vi "Process.vi"(8 "error in":errorcluster, 11 "Inst.TC":refnum<class "Inst.TC.lvclass">) -> (0 "error out":errorcluster, 3 "Inst.TC out":refnum<class "Inst.TC.lvclass">)   [LabVIEW 2019, in "Inst.TC.lvclass"]
doc: "---------------------------------------------------------------\nJKI State Machine Objects™\nhttp://jki.net/state-machine-objects/\nCopyright (C) 2005-2015, JKI <info@jki.net>\nALL RIGHTS RESERVED"
uses:
  Inst.TC.lvclass
  <vilib>/JKI/JKI SMO/SMO/SMO.lvclass
  <userlib>/LevyLab/RemoteControl/RemoteControl/Typedefs/Message--Cluster.ctl
  <userlib>/LevyLab/RemoteControl/RemoteControl/RemoteControl.lvclass
  Typedefs/PrivateEvents--Inst.TC.MessageToProcess.ctl
  C:/Program Files/National Instruments/LabVIEW 2019/user.lib/LevyLab/Instrument Framework/Instrument Types/Cryostat/Instrument.Cryostat.lvclass
  C:/Program Files/National Instruments/LabVIEW 2019/user.lib/LevyLab/Instrument Framework/Instrument/Instrument.lvclass
  C:/Program Files/National Instruments/LabVIEW 2019/vi.lib/JKI/JKI SMO/SMO/SMO.lvclass
  <userlib>/LevyLab/Instrument Framework/Instrument/Instrument.lvclass
  <userlib>/LevyLab/Instrument Framework/Instrument Types/Cryostat/Instrument.Cryostat.lvclass
  <userlib>/LevyLab/Instrument Framework/Instrument/API/Instrument.sendMessageToProcess (variant).vi
  <userlib>/LevyLab/Debug/Debug.lvlib
panel:
  out "Status":string
  out "State History":string
  # "Inst.TC"
  # "Inst.TC"
  # "For instructions on how to use the JKI State Machine Objects, examples and video tutorials, visit:\nhttp://jki.net/state-machine-objects/\n\nJKI State Machine Objects™\nhttp://jki.net/state-machine-objects/\nCopyright (C) 2005-2015, JKI <info@jki.net>\nALL RIGHTS RESERVED"
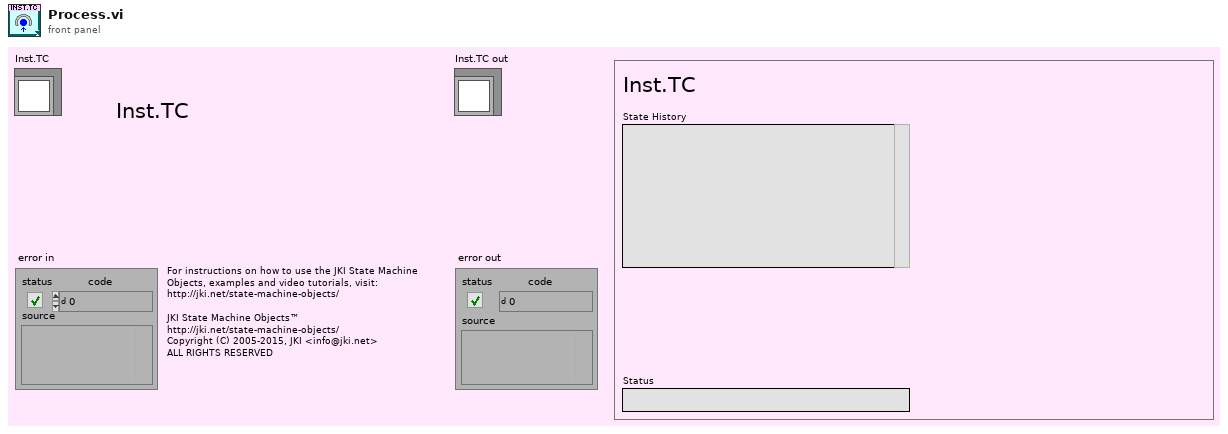
[diagram p1: front panel]
types:
  T1 = enum32{"invalid app kind", "Development System", "Run Time System", "Student Edition", "Embedded LabVIEW", "Evaluation", "Custom"}
  T2 = enum32{"Invalid", "Standard", "Closed", "Hidden", "Minimized", "Maximized"}
  T3 = typedef "RemoteControl.lvlib/RemoteControl.lvclass/Message--Cluster.ctl" = cluster{"Command":string, "Data":variant, "ID":string, "error":errorcluster}
  T4 = typedef "Inst.TC.lvclass/PrivateEvents--Inst.TC.MessageToProcess.ctl" = cluster{"Message":T3}
  T5 = cluster{"Core":cluster{"Current VI Reference":refnum<vi>, "Close Panel on Exit?":bool, "Last Error":cluster{"error":errorcluster, "previous state":string, "remaining states":string}, "Shutdown?":bool}, "SMO":refnum<class "Inst.TC.lvclass">, "Running Step":i32, "sequence":string[], "MessageToProcess":T4}
  T6 = cluster{"Current VI Reference":refnum<vi>, "Close Panel on Exit?":bool, "Last Error":cluster{"error":errorcluster, "previous state":string, "remaining states":string}, "Shutdown?":bool}
  T7 = typedef "SMO.lvclass/Protected Events.ctl" = cluster{"StopProcesses":refnum<user-event>, "AbortProcesses":refnum<user-event>, "Config Changed":refnum<user-event>, "Dependency":refnum<user-event>}
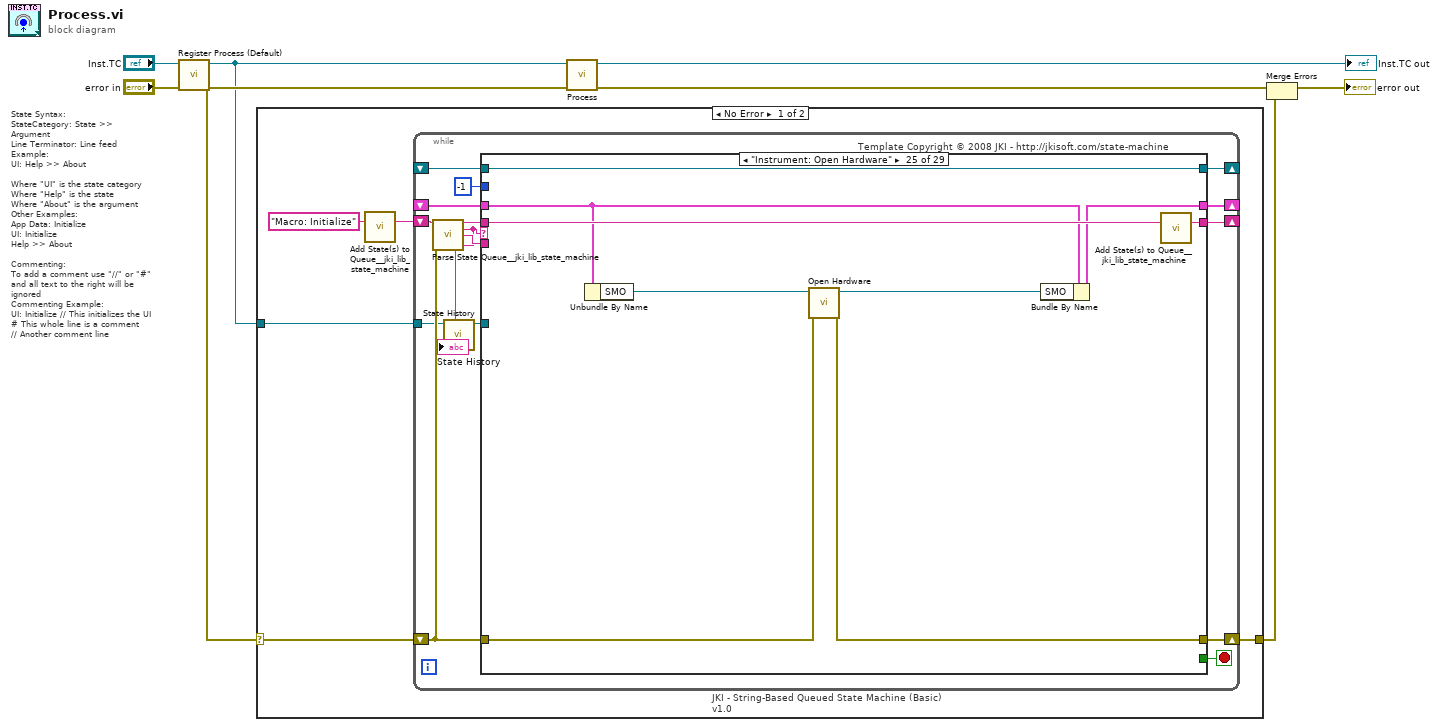
[diagram p0: block diagram]
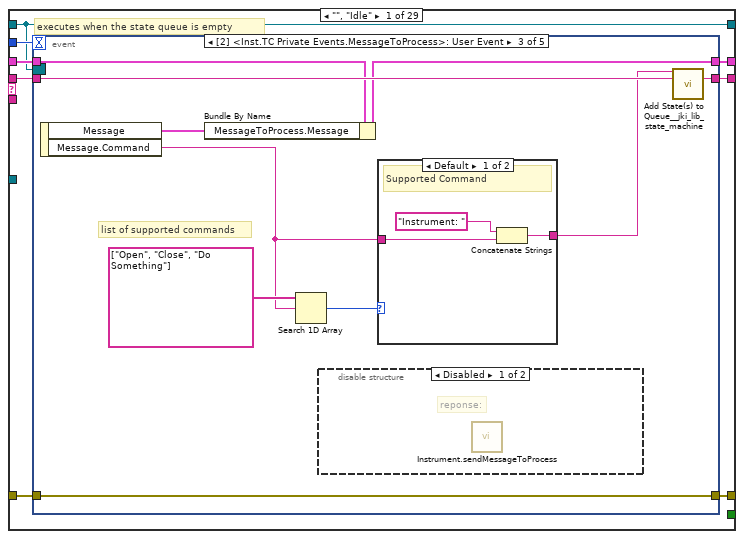
[diagram p2: hidden frame]
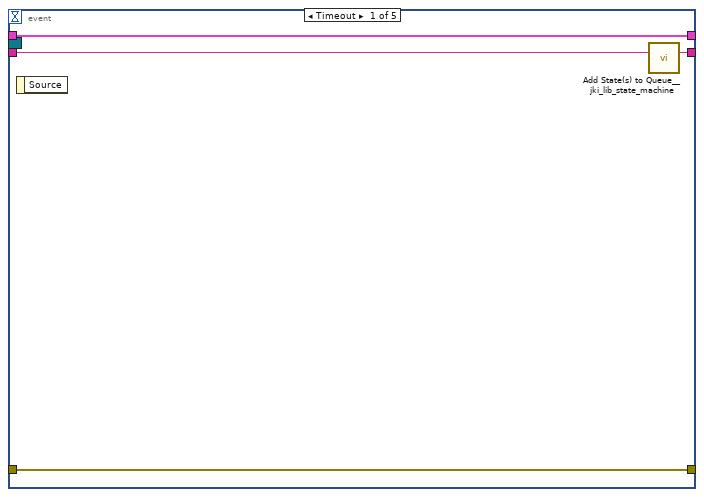
[diagram p3: hidden frame]
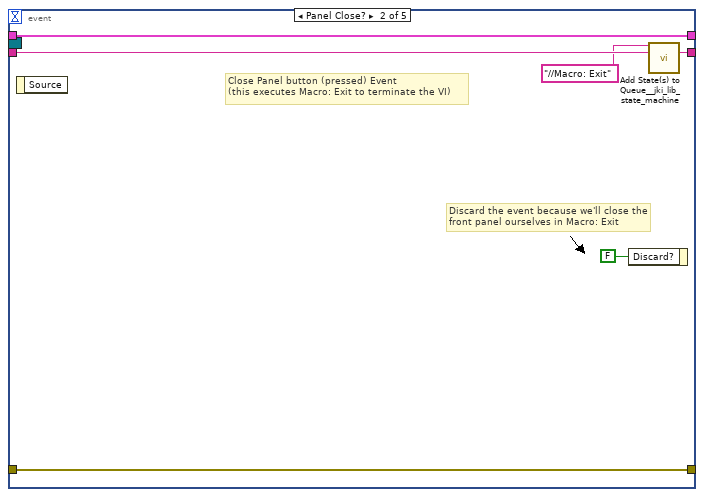
[diagram p4: hidden frame]
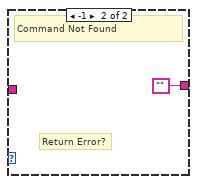
[diagram p6: hidden frame]
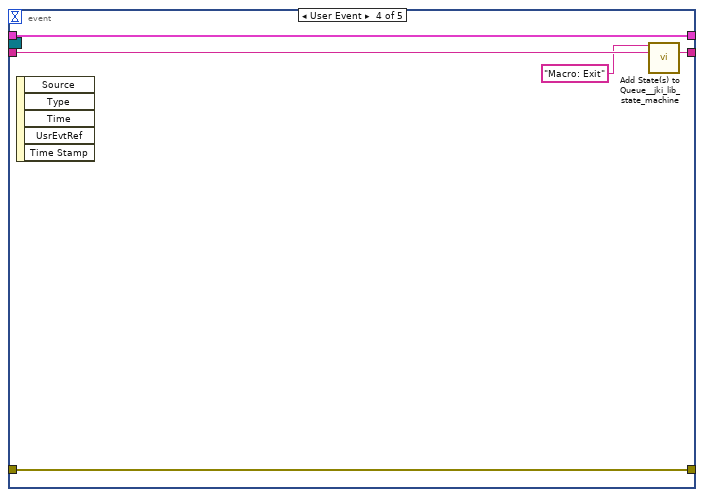
[diagram p7: hidden frame]
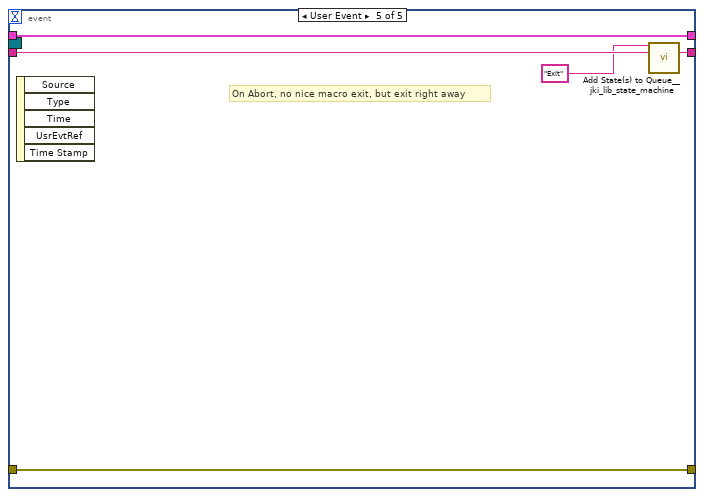
[diagram p8: hidden frame]
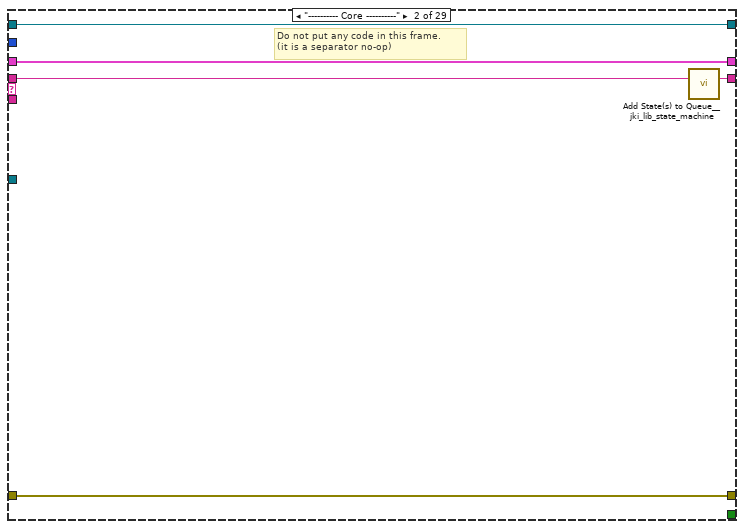
[diagram p9: hidden frame]
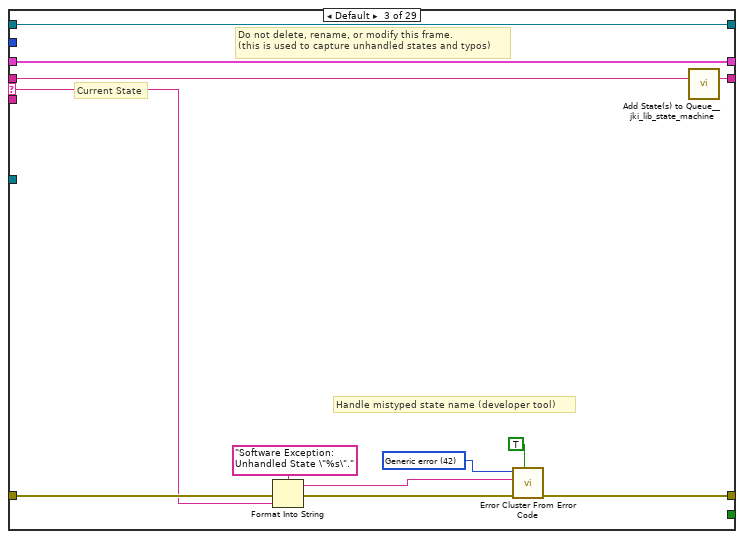
[diagram p10: hidden frame]
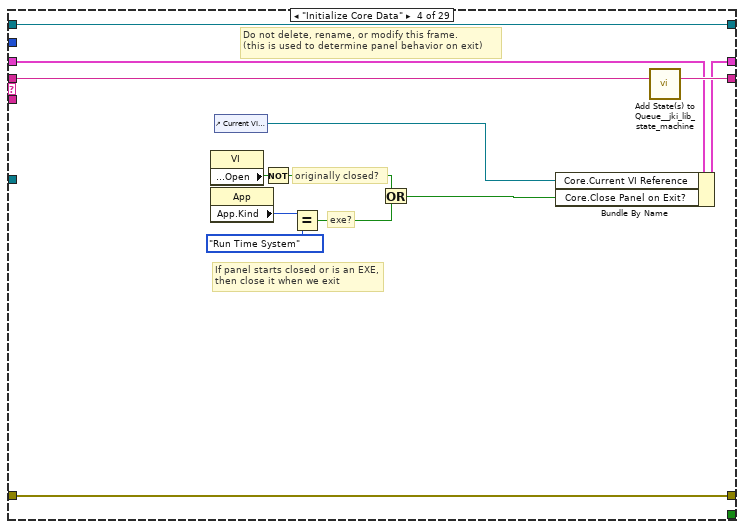
[diagram p11: hidden frame]
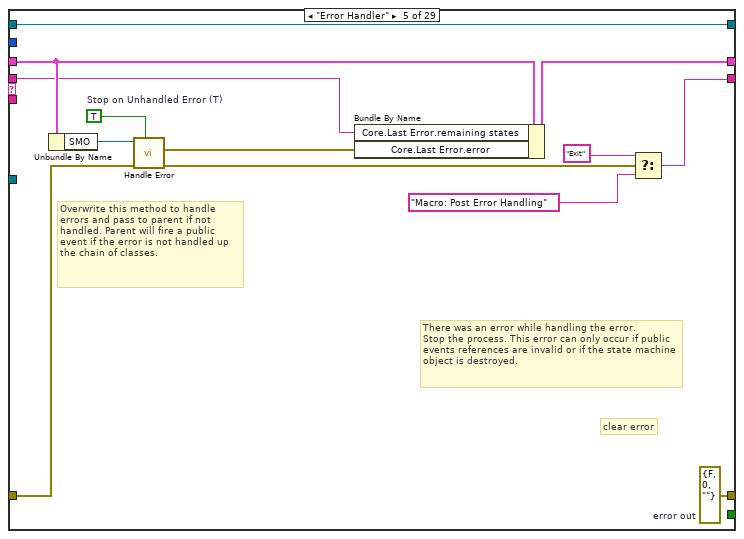
[diagram p12: hidden frame]
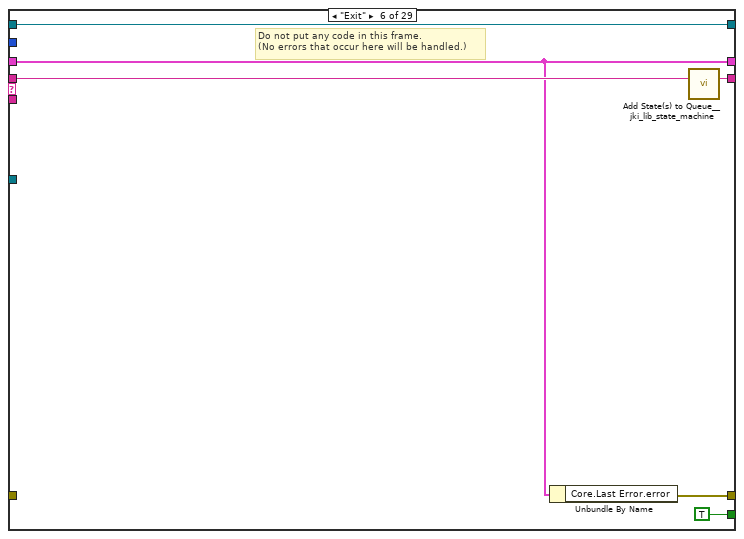
[diagram p13: hidden frame]
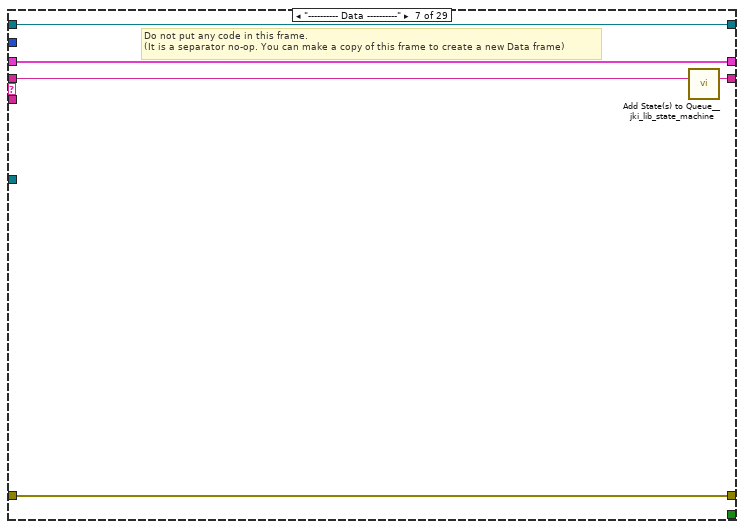
[diagram p14: hidden frame]
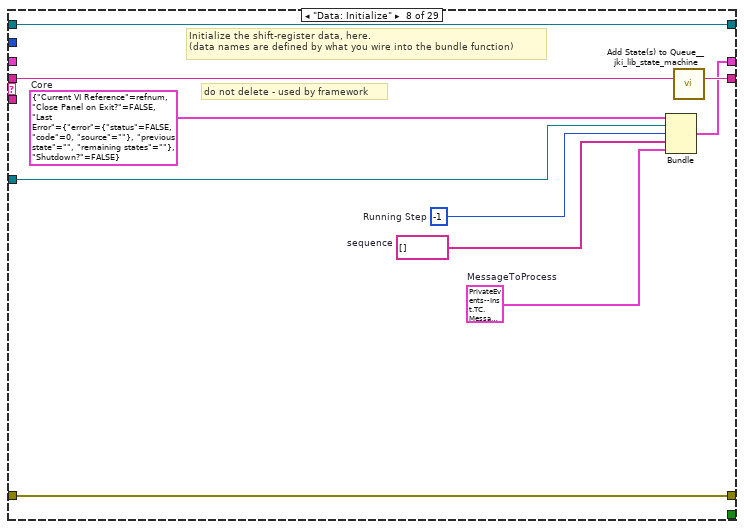
[diagram p15: hidden frame]
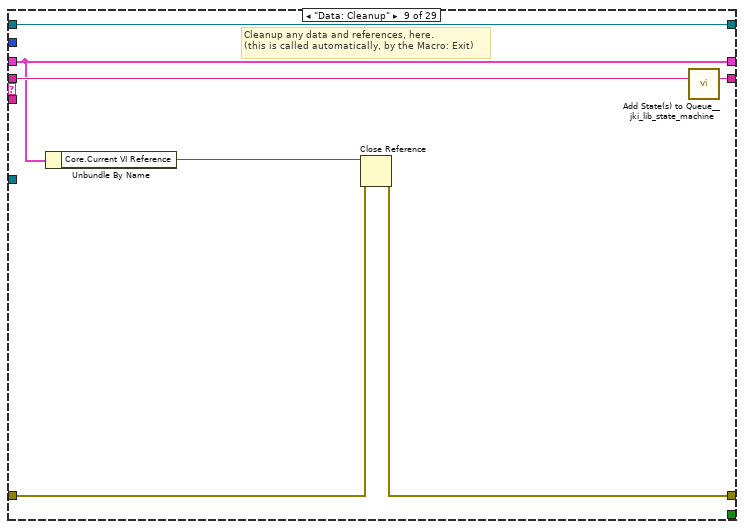
[diagram p16: hidden frame]
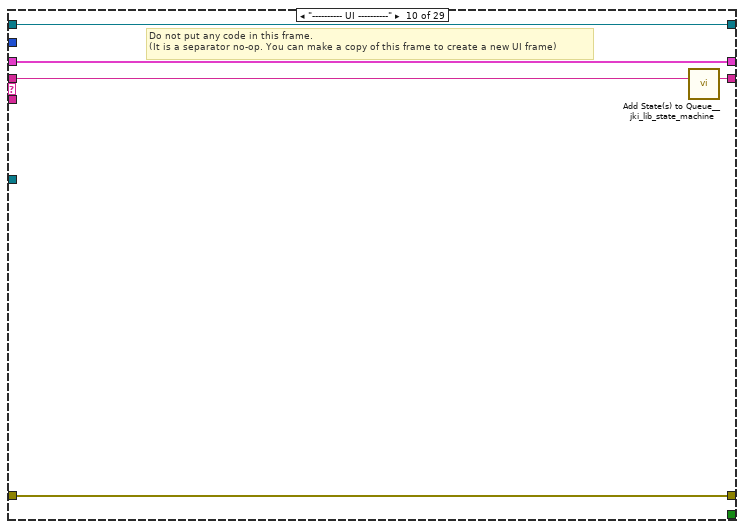
[diagram p17: hidden frame]
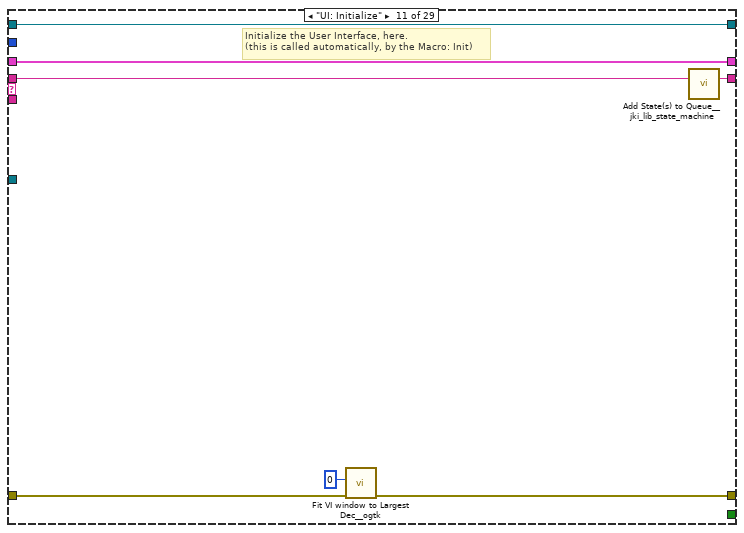
[diagram p18: hidden frame]
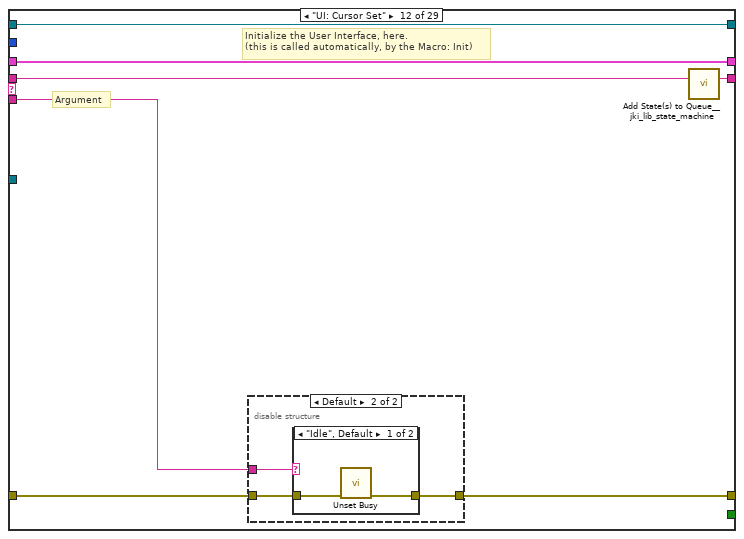
[diagram p19: hidden frame]
diagram:
  # "State Syntax:\nStateCategory: State >> Argument\nLine Terminator: Line feed\nExample:\nUI: Help >> About\n\nWhere \"UI\" is the state category\nWhere \"Help\" is the state\nWhere \"About\" is the argument\nOther Examples:\nApp Data: Initialize\nUI: Initialize\nHelp >> About\n\nCommenting:\nTo add a comment use \"//\" or \"#\" and all text to the right will be ignored\nCommenting Example:\nUI: Initialize // This initializes the UI\n# This whole line is a comment\n// Another comment line"
  n1 = call <vilib>:"Register Process (Default).vi"("error in (no error)"="error in", "SMO"="Inst.TC") -> ("error out"=w5:errorcluster, "SelfRef"=w4:refnum<class "Inst.TC.lvclass">)  [unwired: 8 in]
  n2 = case shown="No Error" w5 {
    selector: w5 -> [w10 w379]
    tunnel: w4 -> [w11 _]
    tunnel: [w9 w379] -> w1
    frame No Error {
      n3 = call <vilib>:"Add State(s) to Queue__jki_lib_state_machine.vi"("State(s) in (\"\")"="Macro: Initialize") -> ("States Out"=w13:string)  [unwired: 14 in]
      n4 = while "JKI - String-Based Queued State Machine (Basic) v1.0" {
        shift-right: [w23] -> _
        shift-left: _ -> [w22]
        shift-right: [w26] -> w9
        shift-left: w10 -> [w20]
        shift-right: [w25] -> _
        shift-left: w13 -> [w27]
        tunnel: w11 -> [w14]
        shift-right: [w19] -> _
        shift-left: _ -> [w18]
        stop <- w24 stop-if-true
        # "Template Copyright © 2008 JKI - http://jkisoft.com/state-machine"
        n5 = call <vilib>:"Parse State Queue__jki_lib_state_machine.vi"("State Queue"=w27, "Error In (no error)"=w20) -> ("Remaining States"=w29:string, "Current State"=w17:string, "Arguments"=w28:string)  [unwired: 11 in]
        n6 = call <userlib>:"State History.vi"("Current State"=w17, "SMO"=w14) -> ("SMO"=w15:refnum<class "Inst.TC.lvclass">, "History"=→"State History":string)  [unwired: 8 in]
        n7 = case shown="\"Instrument: Open Hardware\"" w17 {
          selector: w17 -> [_ _ w78 _ _ _ _ _ _ _ _ _ _ _ _ _ _ _ _ _ _ _ _ _ _ _ _ _ _]
          tunnel: w29 -> [w37 w76 w82 w101 w106 w120 w125 w135 w142 w147 w154 w161 w177 w209 w228 w240 w261 w283 w288 w299 w304 w317 w323 w330 w339 w348 w353 w359 w378]
          tunnel: w28 -> [_ _ _ _ _ _ _ _ _ _ _ w155 w171 _ _ _ _ _ _ _ _ _ _ _ _ _ _ w354 w362]
          tunnel: w22 -> [w35 w73 w80 w92 w110 w116 w122 _ w137 w144 w152 w159 w173 w206 w225 w230 w251 w264 w285 w296 w301 w310 w321 w325 w335 w344 w349 w355 w368]
          tunnel: [w34 w74 w84 w98 w111 w115 w123 w127 w138 w145 w149 w156 w174 w207 w213 w238 w259 w266 w286 w290 w302 w313 w319 w327 w332 w341 w350 w356 w370] -> w26
          tunnel: w20 -> [w33 w74 w83 w98 w112 _ w123 w127 w139 w145 w148 w157 w175 w207 w217 w238 w259 w267 w286 w291 w302 w307 w319 w327 w331 w340 w350 w356 w364]
          tunnel: [w36 w75 w81 w100 w102 w119 w124 w134 w141 w146 w153 w160 w176 w208 w227 w239 w260 w282 w287 w298 w303 w316 w322 w329 w338 w347 w352 w358 w377] -> w25
          tunnel: [_ _ _ _ _ TRUE _ _ _ _ _ _ _ _ _ _ _ _ _ _ _ _ _ _ _ _ _ _ _] -> w24
          tunnel: [w32 w73 w80 w99 w109 w116 w122 w133 w137 w144 w152 w159 w173 w206 w225 w231 w252 w264 w285 w296 w301 w310 w321 w326 w336 w345 w349 w355 w367] -> w23
          tunnel: -1 ("Timeout") -> [w31 _ _ _ _ _ _ _ _ _ _ _ _ _ _ _ _ _ _ _ _ _ _ _ _ _ _ _ _]
          tunnel: w15 -> [_ _ _ _ _ _ _ w128 _ _ _ _ _ _ w221 _ _ w263 _ _ _ _ _ _ _ _ _ _ _]
          tunnel: [w30 w72 w77 w89 w114 w117 w121 w132 w136 w143 w151 w158 w170 w205 w226 w237 w258 w277 w284 w297 w300 w315 w320 w328 w337 w346 w351 w357 w376] -> w19
          tunnel: w18 -> [w30 w72 w77 w89 w114 w117 w121 w132 w136 w143 w151 w158 w170 w205 w226 w237 w258 w277 w284 w297 w300 _ w320 w328 w337 w346 w351 w357 w376]
          frame "", "Idle" {
            # "executes when the state queue is empty"
            n8 = event shown="[2] <Inst.TC Private Events.MessageToProcess>: User Event" {
              selector: w30 -> [_ _ _ _ _]
              dyn-events: _ -> [_ _ _ _ _]
              timeout: w31 -> [_ _ _ _ _]
              tunnel: w37 -> [w41 w47 w57 w66 w71]
              tunnel: [w40 w46 w56 w65 w70] -> w36
              tunnel: w35 -> [w38 w44 w49 w63 w68]
              tunnel: [w39 w45 w55 w64 w69] -> w34
              tunnel: w33 -> [w39 w45 w55 w64 w69]
              tunnel: [w38 w44 w50 w63 w68] -> w32
              event Timeout {
                n9 = event-data() -> ()  [unwired: 1 in, 1 out]
                n10 = call <vilib>:"Add State(s) to Queue__jki_lib_state_machine.vi"("State(s) in (\"\")"=w41) -> ("States Out"=w40:string)  [unwired: 14 in]
              }
              event Panel Close? {
                # "Discard the event because we'll close the front panel ourselves in Macro: Exit"
                # "Close Panel button (pressed) Event\n(this executes Macro: Exit to terminate the VI)"
                n11 = event-data() -> ()  [unwired: 1 in, 1 out]
                n12 = event-data("Discard?"=FALSE) -> ()  [unwired: 1 in, 1 out]
                n13 = call <vilib>:"Add State(s) to Queue__jki_lib_state_machine.vi"("State(s) in Front (\"\")"="//Macro: Exit", "State(s) in (\"\")"=w47) -> ("States Out"=w46:string)  [unwired: 13 in]
              }
              event User Event {
                # "list of supported commands"
                n14 = event-data() -> ("Message"=w48:T3, "Message.Command"=w51:string)  [unwired: 1 in]
                n15 = Bundle By Name(cluster=w49, "MessageToProcess.Message"=w48) -> (w50:T5)
                n16 = Search 1D Array(1D array=string[] ["Open", "Close", "Do Something"], element=w51) -> (index of element=w54:i32)  [unwired: 1 in]
                n17 = disable-structure shown="Disabled" {
                  frame Disabled {
                    # "reponse:"
                    n18 = call-poly <userlib>:"Instrument.sendMessageToProcess.vi"() -> ()  [unwired: 10 in, 2 out]
                  }
                  frame Enabled {
                  }
                }
                n19 = case shown="Default" w54 {
                  tunnel: [w60 "" ("Empty String Constant")] -> w52
                  tunnel: w51 -> [w59 _]
                  frame Default {
                    # "Supported Command"
                    n20 = Concatenate Strings("Instrument: ", w59) -> (w60:string)
                  }
                  frame -1 {
                    # "Return Error?"
                    # "Command Not Found"
                  }
                }
                n21 = call <vilib>:"Add State(s) to Queue__jki_lib_state_machine.vi"("State(s) in Front (\"\")"=w52, "State(s) in (\"\")"=w57) -> ("States Out"=w56:string)  [unwired: 13 in]
              }
              event User Event {
                n22 = event-data() -> ()  [unwired: 1 in, 5 out]
                n23 = call <vilib>:"Add State(s) to Queue__jki_lib_state_machine.vi"("State(s) in Front (\"\")"="Macro: Exit", "State(s) in (\"\")"=w66) -> ("States Out"=w65:string)  [unwired: 13 in]
              }
              event User Event {
                # "On Abort, no nice macro exit, but exit right away"
                n24 = event-data() -> ()  [unwired: 1 in, 5 out]
                n25 = call <vilib>:"Add State(s) to Queue__jki_lib_state_machine.vi"("State(s) in Front (\"\")"="Exit", "State(s) in (\"\")"=w71) -> ("States Out"=w70:string)  [unwired: 13 in]
              }
            }
          }
          frame "---------- Core ----------" {
            # "Do not put any code in this frame.\n(it is a separator no-op)"
            n26 = call <vilib>:"Add State(s) to Queue__jki_lib_state_machine.vi"("State(s) in (\"\")"=w76) -> ("States Out"=w75:string)  [unwired: 14 in]
          }
          frame Default {
            w87 = 42 items=["No error", "Argument error", "Memory is full", "Out of zone", "End of file", "File already open", "Generic file I/O error", "File not found", "File permission error", "Disk is full", "Duplicate path", "Too many files open", "System feature not enabled", "Resource file not found", "Cannot add resource", "Resource not found", "Image not found", "Image memory error", "Pen does not exist", "Config type invalid", "Config token not found", "Config parse error", "Config memory error", "Bad external code format", "Bad external code offset", "External code not present", "Null window", "Destroy window error", "Null menu", "Print aborted", "Bad print record", "Print driver error", "Windows error during printing", "Memory error during printing", "Print dialog error", "Generic print error", "Invalid device refnum", "Device not found", "Device parameter error", "Device unit error", "Cannot open device", "Device call aborted", "Generic error", "Cancelled by user", "Object ID too low", "Object ID too high", "Object not in heap", "Unknown heap", "Unknown object (invalid DefProc)", "Unknown object (DefProc not in table)", "Message out of range", "Invalid (null) method", "Unknown message", "Manager call not supported", "Bad address", "Network operation in progress", "Network operation timed out", "Connection is busy", "Network attribute not supported", "Network error", "Address in use", "System out of memory", "Connection aborted", "Connection refused", "Not connected", "Already connected", "Connection closed", "Initialization error (interapplication manager)", "Bad occurrence", "Wait on unbound occurrence handler", "Occurrence queue overflow", "Datalog type conflict", "Unused", "Unrecognized type (interapplication manager)", "Memory corrupt", "Failed to make temporary DLL", "Old CIN version", "Drag socket not found", "Failed to load drop-object", "Failed to register OLE object", "Failed to release OLE object", "Format specifier type mismatch", "Unknown format specifier", "Too few format specifiers", "Too many format specifiers", "Scan failed", "Newer CIN version", "Error converting to variant", "Runtime menu error", "Password tampered", "Variant attribute not found", "Incompatible variant data type", "Event data is not available", "Event Store is not present", "Occurrence is not found", "Event Queue is not created", "Event info is not available", "Refnum passed is NULL", "Error retrieving Class GUID", "Error retrieving CoClass GUID", "Error retrieving TypeLib GUID.", "Bad built application magic bytes.", "Specific driver is different from the specific driver associated with the Logical Name.", "There is no session opened to the class driver.", "Max Error", "MAX - Error with config objects", "MAX - Error loading configuration", "MAX - Group not supported"]
            # "Current State"
            # "Do not delete, rename, or modify this frame.\n(this is used to capture unhandled states and typos)"
            # "Handle mistyped state name (developer tool)"
            n27 = Format Into String(format string="Software Exception: Unhandled State \"%s\"." ("message"), error in=w83, w78) -> (resulting string=w86:string, error out=w85:errorcluster)  [unwired: 1 in]
            n28 = call <vilib>:"Error Cluster From Error Code.vi"("show call chain? (False)"=TRUE, "error in (no error)"=w85, "error message (\"\")"=w86, "error code (0)"=w87) -> ("error out"=w84:errorcluster)  [unwired: 5 in]
            n29 = call <vilib>:"Add State(s) to Queue__jki_lib_state_machine.vi"("State(s) in (\"\")"=w82) -> ("States Out"=w81:string)  [unwired: 14 in]
          }
          frame "Initialize Core Data" {
            # "Do not delete, rename, or modify this frame.\n(this is used to determine panel behavior on exit)"
            # "originally closed?"
            # "exe?"
            # "If panel starts closed or is an EXE, then close it when we exit"
            n30 = property class="VI"() -> ("Front Panel.Open"=w97:bool)  [unwired: 2 in, 2 out]
            n31 = property class="App"() -> ("App.Kind"=w96:T1)  [unwired: 2 in, 2 out]
            n32 = control-ref of="Current VI Reference"() -> (w90:refnum<vi>)
            n33 = Not(x=w97) -> (.not. x?=w94:bool)
            n34 = Equal?(x=w96, y=T1."Run Time System" ("Application:Kind")) -> (x = y?=w93:bool)
            n35 = Or(x=w94, y=w93) -> (x .or. y?=w91:bool)
            n36 = Bundle By Name(cluster=w92, "Core.Current VI Reference"=w90, "Core.Close Panel on Exit?"=w91) -> (w99:T5)
            n37 = call <vilib>:"Add State(s) to Queue__jki_lib_state_machine.vi"("State(s) in (\"\")"=w101) -> ("States Out"=w100:string)  [unwired: 14 in]
          }
          frame "Error Handler" {
            w107 = TRUE  # Stop on Unhandled Error (T)
            w111 = errorcluster {"status"=FALSE, "code"=0, "source"=""}  # error out
            # "clear error"
            # "There was an error while handling the error.\nStop the process. This error can only occur if public events references are invalid or if the state machine object is destroyed."
            # "Overwrite this method to handle errors and pass to parent if not handled. Parent will fire a public event if the error is not handled up the chain of classes."
            n38 = Unbundle By Name(w110) -> ("SMO"=w113:refnum<class "Inst.TC.lvclass">)
            n39 = call-dynamic "Handle Error.vi"("Stop on Unhandled Error (T)"=w107, "error in"=w112, "SMO"=w113) -> ("handling error"=w103:errorcluster, "Unhandled error"=w108:errorcluster)  [unwired: 6 in, 1 out]
            n40 = Bundle By Name(cluster=w110, "Core.Last Error.remaining states"=w106, "Core.Last Error.error"=w108) -> (w109:T5)
            n41 = Select(t="Exit", s=w103, f="Macro: Post Error Handling") -> (s? t:f=w102:string)
          }
          frame "Exit" {
            # "Do not put any code in this frame.\n(No errors that occur here will be handled.)"
            n42 = Unbundle By Name(w116) -> ("Core.Last Error.error"=w115:errorcluster)
            n43 = call <vilib>:"Add State(s) to Queue__jki_lib_state_machine.vi"("State(s) in (\"\")"=w120) -> ("States Out"=w119:string)  [unwired: 14 in]
          }
          frame "---------- Data ----------" {
            # "Do not put any code in this frame.\n(It is a separator no-op. You can make a copy of this frame to create a new Data frame)"
            n44 = call <vilib>:"Add State(s) to Queue__jki_lib_state_machine.vi"("State(s) in (\"\")"=w125) -> ("States Out"=w124:string)  [unwired: 14 in]
          }
          frame "Data: Initialize" {
            w126 = T4 {"Message"={"Command"="", "Data"=variant(string ""), "ID"="", "error"={"status"=FALSE, "code"=0, "source"=""}}}  # MessageToProcess
            w129 = string[] []  # sequence
            w130 = -1  # Running Step
            w131 = T6 {"Current VI Reference"=refnum, "Close Panel on Exit?"=FALSE, "Last Error"={"error"={"status"=FALSE, "code"=0, "source"=""}, "previous state"="", "remaining states"=""}, "Shutdown?"=FALSE}  # Core
            # "do not delete - used by framework"
            # "Initialize the shift-register data, here.\n(data names are defined by what you wire into the bundle function)"
            n45 = Bundle("Core"=w131, "SMO"=w128, "Running Step"=w130, "sequence"=w129, "MessageToProcess"=w126) -> (w133:T5)  [unwired: 1 in]
            n46 = call <vilib>:"Add State(s) to Queue__jki_lib_state_machine.vi"("State(s) in (\"\")"=w135) -> ("States Out"=w134:string)  [unwired: 14 in]
          }
          frame "Data: Cleanup" {
            # "Cleanup any data and references, here.\n(this is called automatically, by the Macro: Exit)"
            n47 = Unbundle By Name(w137) -> ("Core.Current VI Reference"=w140:refnum<vi>)
            n48 = Close Reference(reference=w140, error in (no error)=w139) -> (error out=w138:errorcluster)
            n49 = call <vilib>:"Add State(s) to Queue__jki_lib_state_machine.vi"("State(s) in (\"\")"=w142) -> ("States Out"=w141:string)  [unwired: 14 in]
          }
          frame "---------- UI ----------" {
            # "Do not put any code in this frame.\n(It is a separator no-op. You can make a copy of this frame to create a new UI frame)"
            n50 = call <vilib>:"Add State(s) to Queue__jki_lib_state_machine.vi"("State(s) in (\"\")"=w147) -> ("States Out"=w146:string)  [unwired: 14 in]
          }
          frame "UI: Initialize" {
            # "Initialize the User Interface, here.\n(this is called automatically, by the Macro: Init)"
            n51 = call <userlib>:"Fit VI window to Largest Dec__ogtk.vi"("error in (no error)"=w148, "border spacing (2 px)"=0) -> ("error out"=w149:errorcluster)  [unwired: 4 in, 1 out]
            n52 = call <vilib>:"Add State(s) to Queue__jki_lib_state_machine.vi"("State(s) in (\"\")"=w154) -> ("States Out"=w153:string)  [unwired: 14 in]
          }
          frame "UI: Cursor Set" {
            # "Argument"
            # "Initialize the User Interface, here.\n(this is called automatically, by the Macro: Init)"
            n53 = disable-structure shown="Default" {
              disable-tunnel: w157 -> [w162 w165]
              disable-tunnel: [w162 w164] -> w156
              disable-tunnel: w155 -> [_ w163]
              frame condition #0 {
              }
              frame condition #1 (active) {
                n54 = case shown="\"Idle\", Default" w163 {
                  tunnel: w165 -> [w167 w169]
                  tunnel: [w166 w168] -> w164
                  frame "Idle", Default {
                    n55 = call <vilib>:"Unset Busy.vi"("error in (no error)"=w167) -> ("error out"=w166:errorcluster)  [unwired: 10 in]
                  }
                  frame "Busy" {
                    n56 = call <vilib>:"Set Busy.vi"("error in (no error)"=w169) -> ("error out"=w168:errorcluster)  [unwired: 9 in, 1 out]
                  }
                }
              }
            }
            n57 = call <vilib>:"Add State(s) to Queue__jki_lib_state_machine.vi"("State(s) in (\"\")"=w161) -> ("States Out"=w160:string)  [unwired: 14 in]
          }
          frame "UI: Front Panel State" {
            # "Argument"
            # "Set Front Panel Open or Closed\n(Usage: \"UI: Front Panel State >> Open|Close\")"
            n58 = Unbundle By Name(w173) -> ("Core.Current VI Reference"=w172:refnum<vi>)
            n59 = disable-structure shown="TARGET_TYPE==RT" {
              disable-tunnel: w175 -> [w181 w204]
              disable-tunnel: [w180 w204] -> w174
              disable-tunnel: w172 -> [w179 _]
              disable-tunnel: w171 -> [w178 _]
              frame condition #0 (active) {
                n60 = case shown="\"Close\"" w178 {
                  tunnel: w181 -> [w185 w198]
                  tunnel: [w187 w199] -> w180
                  tunnel: w179 -> [w186 w196]
                  frame "Open", Default {
                    n61 = property class="VI"(reference=w186, error in=w185) -> (reference out=w183:refnum<vi>, error out=w184:errorcluster, "FP.State"=w182:T2)
                    n62 = case shown="\"Closed\"" w182 {
                      tunnel: [w190 w193] -> w187
                      tunnel: w184 -> [w189 w193]
                      tunnel: w183 -> [w188 _]
                      frame "Closed" {
                        n63 = invoke class="VI" method="FP.Open"(reference=w188, error in=w189, "Activate"=TRUE, "State"=T2."Standard") -> (error out=w190:errorcluster)  [unwired: 1 in, 4 out]
                      }
                      frame Default {
                      }
                    }
                  }
                  frame "Close" {
                    n64 = property class="VI"(reference=w196, error in=w198) -> (reference out=w195:refnum<vi>, error out=w197:errorcluster, "FP.State"=w194:T2)
                    n65 = case shown="Default" w194 {
                      tunnel: [w200 w203] -> w199
                      tunnel: w197 -> [w200 w202]
                      tunnel: w195 -> [_ w201]
                      frame "Invalid", "Closed" {
                      }
                      frame Default {
                        n66 = invoke class="VI" method="FP.Close"(reference=w201, error in=w202) -> (error out=w203:errorcluster)  [unwired: 1 in, 2 out]
                      }
                    }
                  }
                }
              }
              frame condition #1 {
              }
            }
            n67 = call <vilib>:"Add State(s) to Queue__jki_lib_state_machine.vi"("State(s) in (\"\")"=w177) -> ("States Out"=w176:string)  [unwired: 14 in]
          }
          frame "---------- Macro ----------" {
            # "Do not put any code in this frame.\n(It is a separator no-op. You can make a copy of this frame to create a new Macro frame)"
            n68 = call <vilib>:"Add State(s) to Queue__jki_lib_state_machine.vi"("State(s) in (\"\")"=w209) -> ("States Out"=w208:string)  [unwired: 14 in]
          }
          frame "Macro: Initialize" {
            # "Initialization Macro\n(This is called once, when the VI starts)"
            n69 = call-dynamic "Read Debug Mode.vi"("error in (no error)"=w217, "Instrument in"=w221) -> ("error out"=w216:errorcluster, "Debug Mode?"=w218:bool)  [unwired: 7 in, 1 out]
            n70 = call <userlib>:"Wait (ms)__ogtk.vi"("error in (no error)"=w216, "milliseconds to wait"=u32 0) -> ("error out"=w213:errorcluster)  [unwired: 8 in, 1 out]
            n71 = Select(t="Open", s=w218, f="Close") -> (s? t:f=w214:string)
            n72 = Format Into String(format string="UI: Initialize\nUI: Front Panel State >> %s\nInstrument: Open Hardware", initial string="", w214) -> (resulting string=w215:string)  [unwired: 1 in, 1 out]
            n73 = call <vilib>:"Add State(s) to Queue__jki_lib_state_machine.vi"("State(s) in Front (\"\")"="Data: Initialize\nInitialize Core Data\nEvents: Register", "State(s) in (\"\")"="Process: Sync", "State(s) at Back (\"\")"=w215) -> ("States Out"=w223:string)  [unwired: 12 in]
            n74 = call <vilib>:"Add State(s) to Queue__jki_lib_state_machine.vi"("State(s) in Front (\"\")"=w223, "State(s) in (\"\")"=w228) -> ("States Out"=w227:string)  [unwired: 13 in]
          }
          frame "Macro: Post Error Handling" {
            # "Clear Last Error?"
            n75 = Unbundle By Name(w230) -> ("Core.Last Error.remaining states"=w232:string, "Core.Shutdown?"=w233:bool)
            n76 = Unbundle By Name(w230) -> ("Core.Last Error.error"=w236:errorcluster)
            n77 = case shown="False" FALSE {
              tunnel: w236 -> [w244 _]
              tunnel: [w244 _] -> w235
              frame False {
              }
              frame True {
              }
            }
            n78 = case shown="True" w233 {
              tunnel: w232 -> [w241 w243]
              tunnel: [w241 w242] -> w229
              frame False {
                # "These are the remaining states (at the moment the error occured). States can be altered according to business logic."
                # "NOT SHUTTING DOWN"
              }
              frame True {
                # "Developer can decide to alter the states but should be aware that during the shutdown process, there are certain states that must be run for the SMO to properly shut itself (and this process) down. As such, one can add states to perform additional clean-ups, but should append the remaining state to be executed."
                # "SHUTTING DOWN"
                n79 = call <vilib>:"Add State(s) to Queue__jki_lib_state_machine.vi"("State(s) in (\"\")"=w243) -> ("States Out"=w242:string)  [unwired: 14 in]
              }
            }
            n80 = Bundle By Name(cluster=w230, "Core.Last Error.error"=w235) -> (w231:T5)
            n81 = call <vilib>:"Add State(s) to Queue__jki_lib_state_machine.vi"("State(s) in Front (\"\")"=w229, "State(s) in (\"\")"=w240) -> ("States Out"=w239:string)  [unwired: 13 in]
          }
          frame "Macro: Run Sequence" {
            # "0,1,2,3,4,"
            # "5"
            # "Do not put any code in this frame.\n(It is a separator no-op. You can make a copy of this frame to create a new Macro frame)"
            n82 = Unbundle By Name(w251) -> ("sequence"=w247:string[], "Running Step"=w245:i32)
            n83 = Array Size(array=w247) -> (size(s)=w257:i32)
            n84 = Index Array(array=w247, index=w245) -> (element=w246:string)
            n85 = Greater Or Equal?(x=w257, y=w245) -> (x >= y?=w249:bool)
            n86 = Select(t=-1 ("Running Step"), s=w249, f=w245) -> (s? t:f=w256:i32)
            n87 = Bundle By Name(cluster=w251, "Running Step"=w256) -> (w252:T5)
            n88 = Select(t="Sequence: Status >> ...", s=w249, f="Idle //Check Event Structure\nMacro: Run Sequence" ("State(s) at Back (\"\")")) -> (s? t:f=w248:string)
            n89 = call <vilib>:"Add State(s) to Queue__jki_lib_state_machine.vi"("State(s) in Front (\"\")"=w246, "State(s) at Back (\"\")"=w248) -> ("States Out"=w250:string)  [unwired: 13 in]
            n90 = call <vilib>:"Add State(s) to Queue__jki_lib_state_machine.vi"("State(s) in Front (\"\")"=w250, "State(s) in (\"\")"=w261) -> ("States Out"=w260:string)  [unwired: 13 in]
          }
          frame "Macro: Exit" {
            # "Exit Macro\n(This is called once, when the VI exits)"
            n91 = Unbundle By Name(w264) -> ("Core.Close Panel on Exit?"=w281:bool)
            n92 = call-dynamic "Read Debug Mode.vi"("error in (no error)"=w267, "Instrument in"=w263) -> ("error out"=w266:errorcluster, "Debug Mode?"=w265:bool)  [unwired: 7 in, 1 out]
            n93 = Select(t="Open", s=w265, f="Close") -> (s? t:f=w271:string)
            n94 = call <vilib>:"Build State String with Arguments__JKI_lib_State_Machine.vi"("Arguments (\"\")"=w271, "State"="UI: Front Panel State") -> ("State with Arguments"=w268:string)  [unwired: 4 in]
            n95 = Select(t=w268, s=w281, f="" ("Empty String Constant")) -> (s? t:f=w279:string)
            n96 = call <vilib>:"Add State(s) to Queue__jki_lib_state_machine.vi"("State(s) in Front (\"\")"="Data: Cleanup\nEvents: Unregister", "State(s) in (\"\")"="Process: Sync", "State(s) at Back (\"\")"="Exit") -> ("States Out"=w274:string)  [unwired: 12 in]
            n97 = call <vilib>:"Add State(s) to Queue__jki_lib_state_machine.vi"("State(s) in Front (\"\")"="Instrument: Close Hardware", "State(s) in (\"\")"=w279, "State(s) at Back (\"\")"=w274) -> ("States Out"=w278:string)  [unwired: 12 in]
            n98 = call <vilib>:"Add State(s) to Queue__jki_lib_state_machine.vi"("State(s) in Front (\"\")"=w278, "State(s) in (\"\")"=w283) -> ("States Out"=w282:string)  [unwired: 13 in]
          }
          frame "---------- Process ----------" {
            # "Template Separator\n(You can make a copy of, or modify, this frame)"
            n99 = call <vilib>:"Add State(s) to Queue__jki_lib_state_machine.vi"("State(s) in (\"\")"=w288) -> ("States Out"=w287:string)  [unwired: 14 in]
          }
          frame "Process: Sync" {
            n100 = Unbundle By Name(w296) -> ("SMO"=w292:refnum<class "Inst.TC.lvclass">)
            n101 = call <vilib>:"WaitOnProcessSync.vi"("error in (no error)"=w291, "SMO"=w292) -> ("error out"=w290:errorcluster, "Don't run?"=w295:bool)  [unwired: 7 in, 1 out]
            n102 = Select(t="Data: Cleanup\nEvents: Unregister\nExit", s=w295, f="" ("Empty String Constant")) -> (s? t:f=w289:string)
            n103 = call <vilib>:"Add State(s) to Queue__jki_lib_state_machine.vi"("State(s) in Front (\"\")"=w289, "State(s) in (\"\")"=w299) -> ("States Out"=w298:string)  [unwired: 13 in]
          }
          frame "---------- Events ----------" {
            # "Template Separator\n(You can make a copy of, or modify, this frame)"
            n104 = call <vilib>:"Add State(s) to Queue__jki_lib_state_machine.vi"("State(s) in (\"\")"=w304) -> ("States Out"=w303:string)  [unwired: 14 in]
          }
          frame "Events: Register" {
            n105 = Unbundle By Name(w310) -> ("SMO"=w311:refnum<class "Inst.TC.lvclass">)
            n106 = call <vilib>:"GetProtectedEvents.vi"("SMO"=w311) -> ("error out"=w309:errorcluster, "SMO Protected Events"=w314:T7, "SMO out"=w308:refnum<class "Inst.TC.lvclass">)  [unwired: 8 in]
            n107 = call "Inst.TC.GetPrivateEvents.vi"("Inst.TC in"=w308) -> ("error out"=w305:errorcluster, "Inst.TC Private Events"=w306:cluster{"MessageToProcess":refnum<user-event>})  [unwired: 8 in, 1 out]
            n108 = register-events(w314, w306) -> (reference out=w315:refnum<event-registration>, error out=w312:errorcluster)  [unwired: 2 in]
            n109 = Merge Errors(w312, w305, w309, w307) -> (w313:errorcluster)
            n110 = call <vilib>:"Add State(s) to Queue__jki_lib_state_machine.vi"("State(s) in (\"\")"=w317) -> ("States Out"=w316:string)  [unwired: 14 in]
          }
          frame "Events: Unregister" {
            n111 = Unregister For Events(event registration refnum=w320, error in=w319) -> (error out=w318:errorcluster)
            n112 = call <vilib>:"Clear Errors.vi"("error in (no error)"=w318) -> ()  [unwired: 5 in, 2 out]
            n113 = call <vilib>:"Add State(s) to Queue__jki_lib_state_machine.vi"("State(s) in (\"\")"=w323) -> ("States Out"=w322:string)  [unwired: 14 in]
          }
          frame "---------- Instrument ----------" {
            n114 = Unbundle By Name(w325) -> ("SMO"=w324:refnum<class "Inst.TC.lvclass">)
            n115 = Bundle By Name(cluster=w325, "SMO"=w324) -> (w326:T5)
            n116 = call <vilib>:"Add State(s) to Queue__jki_lib_state_machine.vi"("State(s) in (\"\")"=w330) -> ("States Out"=w329:string)  [unwired: 14 in]
          }
          frame "Instrument: Open Hardware" {
            n117 = Unbundle By Name(w335) -> ("SMO"=w334:refnum<class "Inst.TC.lvclass">)
            n118 = call-dynamic "Open Hardware.vi"("error in (no error)"=w331, "Inst.TC in"=w334) -> ("error out"=w332:errorcluster, "Inst.TC out"=w333:refnum<class "Inst.TC.lvclass">)  [unwired: 8 in]
            n119 = Bundle By Name(cluster=w335, "SMO"=w333) -> (w336:T5)
            n120 = call <vilib>:"Add State(s) to Queue__jki_lib_state_machine.vi"("State(s) in (\"\")"=w339) -> ("States Out"=w338:string)  [unwired: 14 in]
          }
          frame "Instrument: Close Hardware" {
            n121 = Unbundle By Name(w344) -> ("SMO"=w343:refnum<class "Inst.TC.lvclass">)
            n122 = call-dynamic "Close Hardware.vi"("error in (no error)"=w340, "Inst.TC in"=w343) -> ("error out"=w341:errorcluster, "Inst.TC out"=w342:refnum<class "Inst.TC.lvclass">)  [unwired: 8 in]
            n123 = Bundle By Name(cluster=w344, "SMO"=w342) -> (w345:T5)
            n124 = call <vilib>:"Add State(s) to Queue__jki_lib_state_machine.vi"("State(s) in (\"\")"=w348) -> ("States Out"=w347:string)  [unwired: 14 in]
          }
          frame "---------- Sequence ----------" {
            n125 = call <vilib>:"Add State(s) to Queue__jki_lib_state_machine.vi"("State(s) in (\"\")"=w353) -> ("States Out"=w352:string)  [unwired: 14 in]
          }
          frame "Sequence: Status" {
            # "Sequence: Status\n(Use this frame to pass the status to the UI, this VI's UI, etc)"
            n126 = call <vilib>:"Add State(s) to Queue__jki_lib_state_machine.vi"("State(s) in (\"\")"=w359) -> ("States Out"=w358:string)  [unwired: 14 in]
            "Status" <- w354
          }
          frame "Sequence: Wait" {
            # "Sequence: Wait\n(Non-Blocking Wait)"
            # "F = repeat this state. wait\nT = go to next state. don't wait"
            n127 = Unbundle By Name(w368) -> ("Running Step"=w361:i32)
            n128 = call <userlib>:"Wait Logic.vi"("error in (no error)"=w364, "Time"=w362) -> ("error out"=w363:errorcluster, "Status String"=w360:string, "Trigger"=w365:bool)  [unwired: 6 in, 1 out]
            n129 = Increment(x=w361) -> (x+1=w375:i32)
            n130 = Select(t=w375, s=w365, f=w361) -> (s? t:f=w366:i32)
            n131 = Select(t=u32 0, s=w365, f=u32 100 ("milliseconds to wait")) -> (s? t:f=w372:u32)
            n132 = call <userlib>:"Wait (ms)__ogtk.vi"("error in (no error)"=w363, "milliseconds to wait"=w372) -> ("error out"=w370:errorcluster)  [unwired: 8 in, 1 out]
            n133 = Bundle By Name(cluster=w368, "Running Step"=w366) -> (w367:T5)
            n134 = call <vilib>:"Build State String with Arguments__JKI_lib_State_Machine.vi"("Arguments (\"\")"=w360, "State"="Sequence: Status") -> ("State with Arguments"=w369:string)  [unwired: 4 in]
            n135 = call <vilib>:"Add State(s) to Queue__jki_lib_state_machine.vi"("State(s) in Front (\"\")"=w369, "State(s) in (\"\")"=w378) -> ("States Out"=w377:string)  [unwired: 13 in]
          }
        }
      }
    }
    frame Error {
    }
  }
  n136 = call-parent "Process.vi"("error in"=w5, "Instrument"=w4) -> ("error out"=w2:errorcluster, "Instrument out"=→"Inst.TC out":refnum<class "Inst.TC.lvclass">)  [unwired: 8 in]
  n137 = Merge Errors(w2, w1) -> (→"error out":errorcluster)
